vi "SensorGUI_9Feb23.vi"() -> ()   [LabVIEW 2022 SP3]
uses:
  <vilib>/Instr/_visa.llb/VISA Configure Serial Port (Instr).vi
panel:
  out "Sensor 0":i32
  out "Sensor 1":i32
  out "Sensor 2":i32
  out "Sensor 3":i32
  out "Sensor 5":i32
  out "Sensor 4":i32
  out "Sensor 7":i32
  out "Sensor 6":i32
  in  "Record Instantaneous Pressure":bool
  out "Live Plot":i32[][](graph)
  out "Elapsed Iterations":i32
  in  "Log File":path
  in  "Stop VI":bool
  in  "Serial Port":refnum<visa-resource-name>
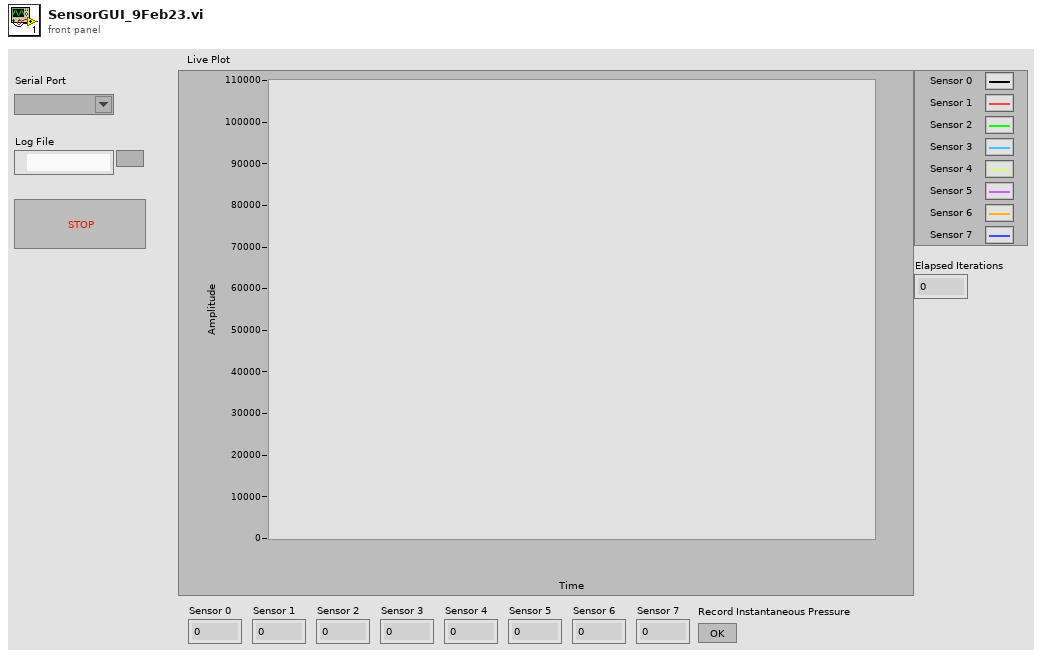
[diagram p1: front panel]
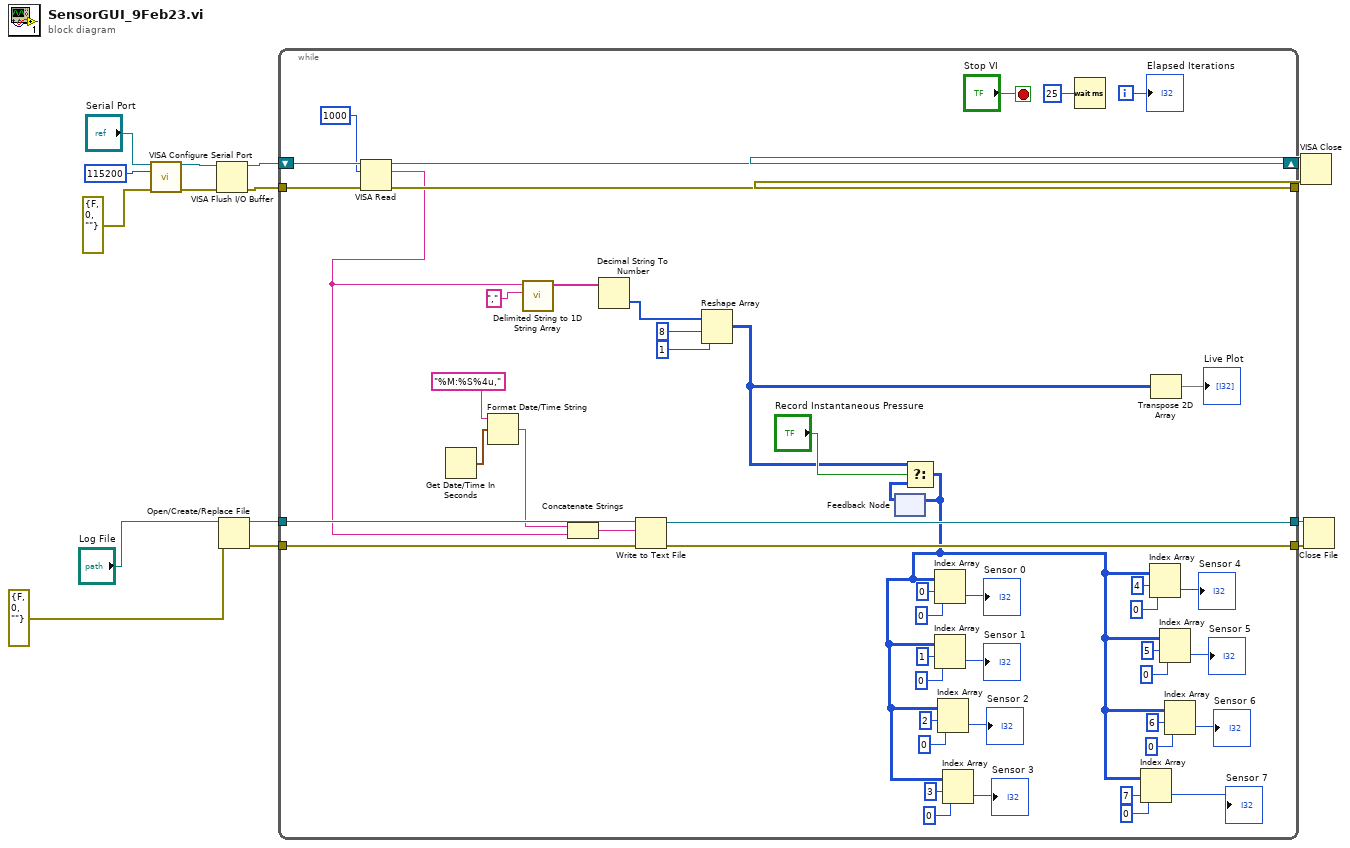
[diagram p0: block diagram]
diagram:
  n1 = call-poly "VISA Configure Serial Port"("VISA resource name"="Serial Port", "baud rate (9600)"=u32 115200, "error in (no error)"=errorcluster {"status"=FALSE, "code"=0, "source"=""}) -> ("VISA resource name out"=w6:refnum<visa-resource-name>, "error out"=w4:errorcluster)  [unwired: 11 in]
  n2 = VISA Flush I/O Buffer(VISA resource name=w6, error in (no error)=w4) -> (VISA resource name out=w5:refnum<visa-resource-name>, error out=w3:errorcluster)  [unwired: 1 in]
  n3 = Open/Create/Replace File(file path (use dialog)="Log File", error in=errorcluster {"status"=FALSE, "code"=0, "source"=""}) -> (refnum out=w10:refnum<file>, error out=w9:errorcluster)  [unwired: 4 in, 1 out]
  n4 = while {
    shift-right: [w65] -> w14
    shift-left: w5 -> [w66]
    tunnel: w3 -> [w62]
    tunnel: [w61] -> w13
    tunnel: w10 -> [w60]
    tunnel: w9 -> [w59]
    tunnel: [w58] -> w8
    tunnel: [w57] -> w7
    i -> [w54]
    stop <- "Stop VI" stop-if-true
    n5 = VISA Read(VISA resource name=w66, byte count=u32 1000, error in (no error)=w62) -> (VISA resource name out=w65:refnum<visa-resource-name>, read buffer=w45:string, error out=w61:errorcluster)  [unwired: 1 out]
    n6 = Get Date/Time In Seconds() -> (seconds since 1Jan1904=w38:timestamp)
    n7 = Format Date/Time String(time format string (%c)="%M:%S%4u,", seconds (now)=w38) -> (date/time string=w46:string)  [unwired: 1 in]
    n8 = call <vilib>:"Delimited String to 1D String Array.vi"("delimiter"=",", "delimited string"=w45) -> ("string array"=w55:string[])  [unwired: 9 in]
    n9 = Concatenate Strings(w46, w45) -> (w47:string)
    n10 = Decimal String To Number(string=w55) -> (number=w53:i32[])  [unwired: 2 in, 1 out]
    n11 = Write to Text File(file (use dialog)=w60, text=w47, error in=w59) -> (refnum out=w58:refnum<file>, error out=w57:errorcluster)  [unwired: 1 in, 1 out]
    n12 = Reshape Array(w53, 8 ("dimension size"), 1 ("dimension size")) -> (w35:i32[][])
    n13 = feedback #1() -> (w36:i32[][])  [unwired: 1 in]
    n14 = Select(t=w35, s="Record Instantaneous Pressure", f=w36) -> (s? t:f=w16:i32[][])
    n15 = feedback-in #1(w16) -> ()
    n16 = Index Array(array=w16, index (row)=0, index (col)=0 ("disabled index (col)")) -> (element=→"Sensor 0":i32)
    n17 = Index Array(array=w16, index (row)=1, index (col)=0 ("disabled index (col)")) -> (element=→"Sensor 1":i32)
    n18 = Index Array(array=w16, index (row)=2, index (col)=0 ("disabled index (col)")) -> (element=→"Sensor 2":i32)
    n19 = Index Array(array=w16, index (row)=3, index (col)=0 ("disabled index (col)")) -> (element=→"Sensor 3":i32)
    n20 = Wait (ms)(milliseconds to wait=u32 25) -> ()  [unwired: 1 out]
    n21 = Index Array(array=w16, index (row)=7, index (col)=0 ("disabled index (col)")) -> (element=→"Sensor 7":i32)
    n22 = Index Array(array=w16, index (row)=4, index (col)=0 ("disabled index (col)")) -> (element=→"Sensor 4":i32)
    n23 = Transpose 2D Array(2D array=w35) -> (transposed array=→"Live Plot":i32[][])
    n24 = Index Array(array=w16, index (row)=5, index (col)=0 ("disabled index (col)")) -> (element=→"Sensor 5":i32)
    n25 = Index Array(array=w16, index (row)=6, index (col)=0 ("disabled index (col)")) -> (element=→"Sensor 6":i32)
    "Elapsed Iterations" <- w54
  }
  n26 = VISA Close(VISA resource name=w14, error in (no error)=w13) -> ()  [unwired: 1 out]
  n27 = Close File(refnum=w8, error in=w7) -> ()  [unwired: 2 out]
